vi "Write COM SELECTED CY.vi"(8 "error in (no error)":errorcluster, 10 "COM SELECTED":refnum<visa-resource-name>, 11 "TI in":refnum<class "CYPRESS.lvclass">) -> (0 "error out":errorcluster, 3 "TI out":refnum<class "CYPRESS.lvclass">)   [LabVIEW 2019, in "CYPRESS.lvclass"]
uses:
  CYPRESS.lvclass
  CYPRESS.lvclass/CYPRESS.ctl
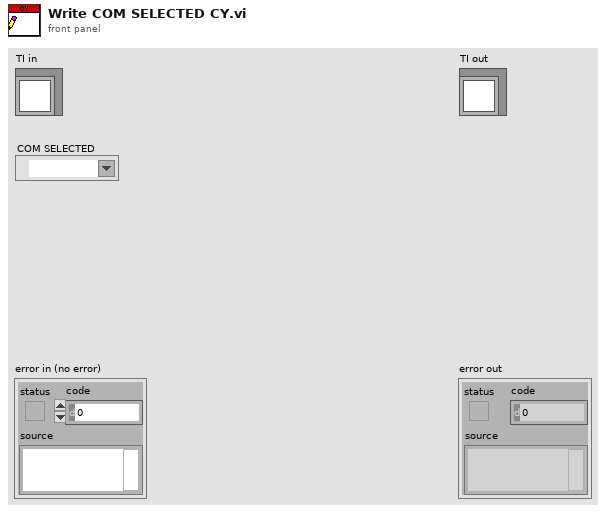
[diagram p1: front panel]
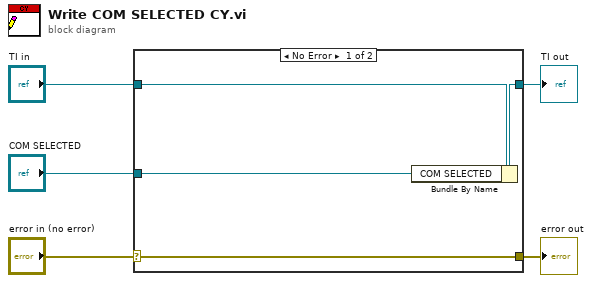
[diagram p0: block diagram]
diagram:
  n1 = case shown="No Error" "error in (no error)" {
    selector: "error in (no error)" -> [w9 w10]
    tunnel: [w9 w10] -> w4
    tunnel: [w7 w11] -> w2
    tunnel: "TI in" -> [w8 w11]
    tunnel: "COM SELECTED" -> [w6 _]
    frame No Error {
      n2 = Bundle By Name(cluster=w8, "COM SELECTED"=w6) -> (w7:refnum<class "CYPRESS.lvclass">)
    }
    frame Error {
    }
  }
  "error out" <- w4
  "TI out" <- w2
